vi "Main.vi"() -> ()   [LabVIEW 2013]
uses:
  <vilib>/myRIO/Instrument Drivers/Onboard IO/I2C/vis/Smart Open.vi
  <vilib>/myRIO/Instrument Drivers/Onboard IO/I2C/vis/Configure.vi
  <vilib>/myRIO/Instrument Drivers/Onboard IO/I2C/vis/Write.vi
  <vilib>/myRIO/Common/Instrument Driver Framework/myRIO v1.0/UART/vis/myRIO v1.0 Close UART.vi
  <vilib>/myRIO/Instrument Drivers/Onboard IO/I2C/vis/Open.vi
  <vilib>/myRIO/Common/Instrument Driver Framework/myRIO v1.0/I2C/vis/myRIO v1.1 Open I2C.vi
  <vilib>/myRIO/Common/Instrument Driver Framework/Utilities/vis/Validate Channels.vi
  <vilib>/myRIO/Common/Instrument Driver Framework/myRIO v1.0/I2C/vis/myRIO v1.0 Reserve I2C.vi
  <vilib>/myRIO/Common/Instrument Driver Framework/myRIO v1.0/I2C/vis/myRIO v1.0 Build MUX Configuration I2C.vi
  <vilib>/myRIO/Common/Instrument Driver Framework/myRIO v1.0/Resource Manager/vis/myRIO v1.0 Reserve Channel List.vi
  <vilib>/myRIO/Common/Instrument Driver Framework/myRIO v1.0/Resource Manager/vis/myRIO v1.0 Create Configuration List.vi
  <vilib>/myRIO/Common/Instrument Driver Framework/myRIO v1.0/Resource Manager/vis/myRIO v1.0 Reserve Channel.vi
  <vilib>/myRIO/Common/Instrument Driver Framework/myRIO v1.0/Resource Manager/vis/myRIO v1.0 Unreserve Channel.vi
  <vilib>/myRIO/Common/Instrument Driver Framework/myRIO v1.0/Resource Manager/vis/myRIO v1.0 Build Mutex Name.vi
  <vilib>/myRIO/Common/Instrument Driver Framework/myRIO v1.0/myRIO v1.1 Open.vi
  <vilib>/Utility/VariantDataType/GetNumericInfo.vi
  <vilib>/Utility/error.llb/Error Cluster From Error Code.vi
  <vilib>/myRIO/Common/Instrument Driver Framework/Utilities/vis/IO Manager.vi
  <vilib>/myRIO/Common/Instrument Driver Framework/Utilities/vis/Configuration Manager.vi
  <vilib>/myRIO/Common/Instrument Driver Framework/myRIO v1.0/Resource Manager/vis/myRIO v1.0 Configure IO.vi
  <vilib>/myRIO/Common/Instrument Driver Framework/myRIO v1.0/myRIO v1.0 Close.vi
  <vilib>/myRIO/Common/Instrument Driver Framework/myRIO v1.0/I2C/vis/myRIO v1.0 Configure I2C.vi
  <vilib>/myRIO/Common/Instrument Driver Framework/myRIO v1.0/I2C/vis/myRIO v1.0 Write I2C.vi
  <vilib>/myRIO/Common/Instrument Driver Framework/Utilities/vis/FPGA Ref Manager.vi
  <vilib>/myRIO/Common/Instrument Driver Framework/myRIO v1.0/myRIO v1.0 Reset FPGA.vi
  <vilib>/myRIO/Instrument Drivers/Utilities/Utilities.lvlib
panel:
  out "LCD display":string
  in  "[ESC]":bool
  # "LCD (I2C) demo"
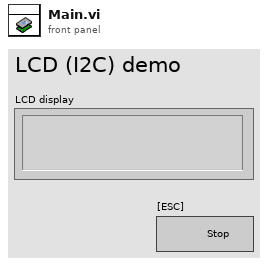
[diagram p1: front panel]
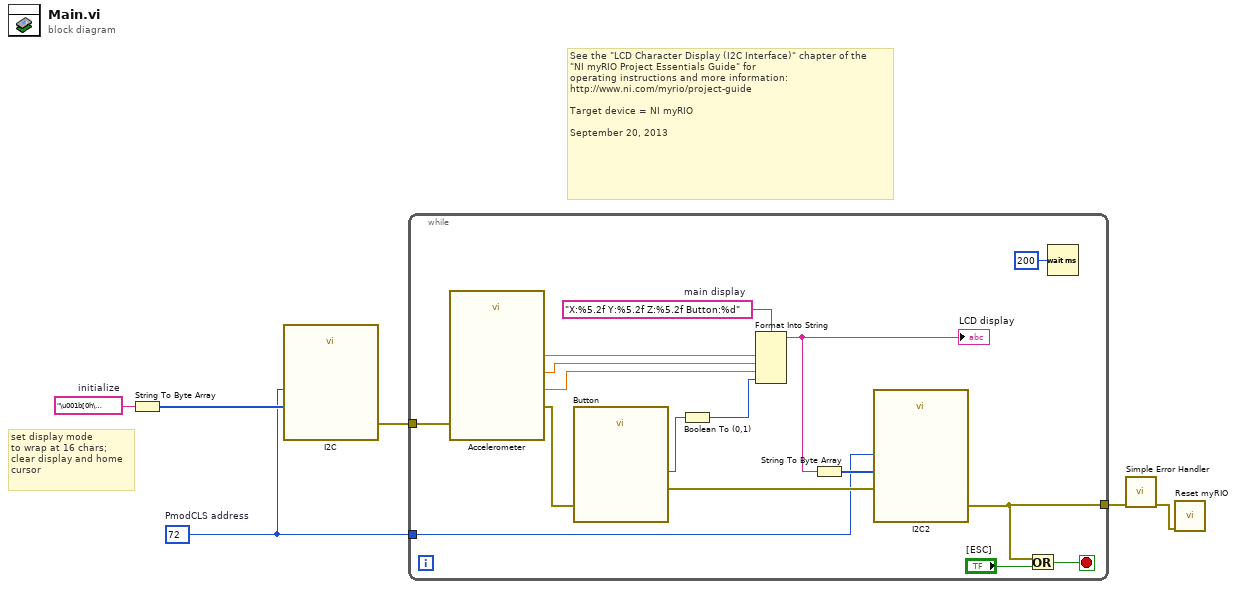
[diagram p0: block diagram]
diagram:
  w1 = u8 72  # PmodCLS address
  w4 = "\u001b[0h\u001b[j"  # initialize
  # "See the \"LCD Character Display (I2C Interface)\" chapter of the\n\"NI myRIO Project Essentials Guide\" for\noperating instructions and more information: \nhttp://www.ni.com/myrio/project-guide\n\nTarget device = NI myRIO\n\nSeptember 20, 2013"
  # "set display mode\nto wrap at 16 chars;\nclear display and home\ncursor"
  n1 = String To Byte Array(string=w4) -> (unsigned byte array=w2:u8[])
  n2 = call "I2C"("Slave Address (7-bit)"=w1, "Bytes to Write"=w2) -> ("error out"=w3:errorcluster)  [unwired: 25 in]
  n3 = while {
    tunnel: [w9] -> w5
    tunnel: w3 -> [w12]
    tunnel: w1 -> [w7]
    stop <- w14 stop-if-true
    w22 = "X:%5.2f Y:%5.2f Z:%5.2f Button:%d"  # main display
    n4 = call "Accelerometer"("error in (no error)"=w12) -> ("X-Axis"=w20:dbl, "Y-Axis"=w19:dbl, "Z-Axis"=w18:dbl, "error out"=w17:errorcluster)  [unwired: 23 in]
    n5 = call "Button"("error in (no error)"=w17) -> ("Value"=w16:bool, "error out"=w8:errorcluster)  [unwired: 25 in]
    n6 = Boolean To (0,1)(Boolean=w16) -> (0, 1=w21:i16)
    n7 = Format Into String "Format Into String"(format string=w22, w20, w19, w18, w21) -> (resulting string=w11:string)  [unwired: 2 in, 1 out]
    "LCD display" <- w11
    n8 = String To Byte Array(string=w11) -> (unsigned byte array=w10:u8[])
    n9 = call "I2C2"("Slave Address (7-bit)"=w7, "Bytes to Write"=w10, "error in (no error)"=w8) -> ("error out"=w9:errorcluster)  [unwired: 24 in]
    n10 = Or(x=w9, y="[ESC]") -> (x .or. y?=w14:bool)
    n11 = Wait (ms)(milliseconds to wait=u32 200) -> ()  [unwired: 1 out]
  }
  n12 = call <vilib>:"Simple Error Handler.vi"("error in (no error)"=w5) -> ("error out"=w6:errorcluster)  [unwired: 4 in, 4 out]
  n13 = call <vilib>:"Reset myRIO.vi"("error in (no error)"=w6) -> ()  [unwired: 10 in, 1 out]
